vi "Pseudo Random Number Generator.vi"(10 "reset":bool, 11 "seed":u16) -> (3 "pseudo random value":u16)   [LabVIEW 2015, in "Engine Simulation Toolkit.lvlib"]
doc: "This VI generates a sequence of pseudo random numbers using a linear feedback shift register algorithm with four taps.\n\nhttp://en.wikipedia.org/wiki/Linear_feedback_shift_register"
uses:
  Engine Simulation Toolkit.lvlib
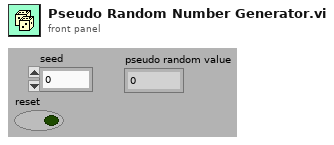
[diagram p1: front panel]
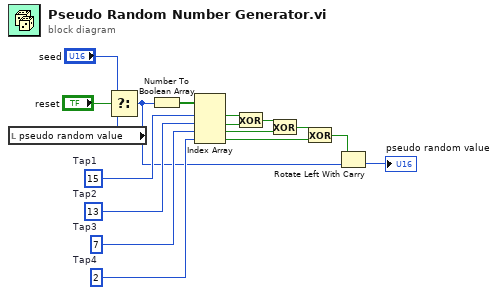
[diagram p0: block diagram]
diagram:
  w8 = 2  # Tap4
  w9 = 7  # Tap3
  w14 = 13  # Tap2
  w15 = 15  # Tap1
  n1 = local read "pseudo random value"() -> (w7:u16)
  n2 = Select(t="seed", s="reset", f=w7) -> (s? t:f=w6:u16)
  n3 = Number To Boolean Array(number=w6) -> (Boolean array=w16:bool[])
  n4 = Index Array(array=w16, index #1=w15, index #2=w14, index #3=w9, index #4=w8) -> (element #1=w13:bool, element #2=w12:bool, element #3=w5:bool, element #4=w11:bool)
  n5 = Exclusive Or(1:w12, 2:w13) -> (0:w10:bool)
  n6 = Exclusive Or(1:w5, 2:w10) -> (0:w4:bool)
  n7 = Exclusive Or(1:w11, 2:w4) -> (0:w3:bool)
  n8 = Rotate Left With Carry(2:w6, 3:w3) -> (0:→"pseudo random value":u16)  [unwired: 1 out]
